vi "Configure Bandwidth.vi"(8 "error in (no error)":errorcluster, 9 "Enable Bandwidth Limit (F: Disable)":bool, 10 "Channel (1: Channel 1)":u16(ring)=1 items=["Channel 1"=1, "Channel 2"=2, "Channel 3"=3, "Channel 4"=4], 11 "VISA resource name":refnum<visa-resource-name>) -> (0 "error out":errorcluster, 3 "VISA resource name out":refnum<visa-resource-name>)   [LabVIEW 2021, in "Siglent SDS 1000 2000 Series.lvlib"]
doc: "Enables or disables the bandwidth-limiting lowpass filter. The command is used to set the bandwidth individually for each channel."
uses:
  <instrlib>/Siglent SDS 1000 2000 Series/Siglent SDS 1000 2000 Series.lvlib
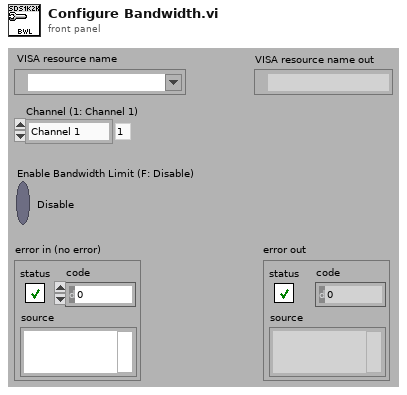
[diagram p1: front panel]
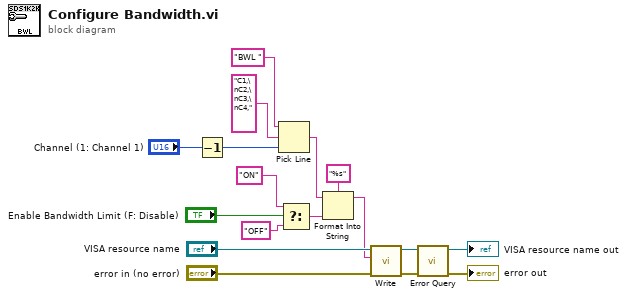
[diagram p0: block diagram]
diagram:
  n1 = Decrement(x="Channel (1: Channel 1)") -> (x-1=w9:u16)
  n2 = Pick Line(string ("")="BWL ", multi-line string="C1,\nC2,\nC3,\nC4,", line index=w9) -> (output string=w6:string)
  n3 = Select(t="ON", s="Enable Bandwidth Limit (F: Disable)", f="OFF") -> (s? t:f=w2:string)
  n4 = Format Into String(format string="%s", initial string=w6, w2) -> (resulting string=w7:string)  [unwired: 1 in, 1 out]
  n5 = call <instrlib>:"Write.vi"("error in (no error)"="error in (no error)", "Write Buffer"=w7, "VISA resource name"="VISA resource name") -> ("error out"=w12:errorcluster, "VISA resource name out"=w13:refnum<visa-resource-name>)  [unwired: 6 in, 1 out]
  n6 = call <instrlib>:"Error Query.vi"("error in (no error)"=w12, "VISA resource name"=w13) -> ("error out"=→"error out":errorcluster, "VISA resource name out"=→"VISA resource name out":refnum<visa-resource-name>)  [unwired: 6 in, 2 out]
